vi "6.vi"   [LabVIEW 2017]
uses:
  <vilib>/myRIO/Instrument Drivers/Onboard IO/PWM/typedefs/PWM Reference.ctl
  <vilib>/myRIO/Common/Instrument Driver Framework/Utilities/typedefs/myRIO Generic Hardware Reference.ctl
  <vilib>/myRIO/Common/Instrument Driver Framework/Utilities/typedefs/Hardware Version Enum.ctl
  <vilib>/myRIO/Common/Instrument Driver Framework/Utilities/typedefs/myRIO v1.0 Reference.ctl
  <vilib>/myRIO/Common/Instrument Driver Framework/Utilities/typedefs/Generic FPGA Reference.ctl
  <vilib>/myRIO/Common/Instrument Driver Framework/myRIO v1.0/PWM/typedefs/PWM Channels Enum.ctl
  <vilib>/myRIO/Instrument Drivers/Onboard IO/PWM/typedefs/PWM Configuration.ctl
  <vilib>/userdefined/High Color/nirio_resource_hc.ctl
  <vilib>/myRIO/Common/Instrument Driver Framework/Utilities/vis/Is FPGA Ref Available.vi
  <vilib>/myRIO/Common/Instrument Driver Framework/myRIO v1.0/PWM/vis/myRIO v1.1 Open PWM.vi
  <vilib>/myRIO/Instrument Drivers/Onboard IO/PWM/vis/Set Duty Cycle and Frequency.vi
  <vilib>/myRIO/Common/Instrument Driver Framework/Utilities/vis/Validate Channels.vi
  <vilib>/myRIO/Common/Instrument Driver Framework/myRIO v1.0/PWM/vis/myRIO v1.0 Reserve PWM.vi
  <vilib>/myRIO/Common/Instrument Driver Framework/myRIO v1.0/PWM/vis/myRIO v1.0 Build MUX Configuration PWM.vi
  <vilib>/myRIO/Common/Instrument Driver Framework/myRIO v1.0/Resource Manager/vis/myRIO v1.0 Reserve Channel List.vi
  <vilib>/myRIO/Common/Instrument Driver Framework/myRIO v1.0/Resource Manager/vis/myRIO v1.0 Create Configuration List.vi
  <vilib>/myRIO/Common/Instrument Driver Framework/myRIO v1.0/Resource Manager/vis/myRIO v1.0 Reserve Channel.vi
  <vilib>/myRIO/Common/Instrument Driver Framework/myRIO v1.0/Resource Manager/vis/myRIO v1.0 Unreserve Channel.vi
  <vilib>/myRIO/Common/Instrument Driver Framework/myRIO v1.0/Resource Manager/vis/myRIO v1.0 Build Mutex Name.vi
  <vilib>/Utility/VariantDataType/GetNumericInfo.vi
  <vilib>/Utility/error.llb/Error Cluster From Error Code.vi
  <vilib>/myRIO/Common/Instrument Driver Framework/myRIO v1.0/myRIO v1.1 Open.vi
  <vilib>/myRIO/Common/Instrument Driver Framework/Utilities/vis/IO Manager.vi
  <vilib>/myRIO/Common/Instrument Driver Framework/Utilities/vis/Configuration Manager.vi
  <vilib>/myRIO/Common/Instrument Driver Framework/myRIO v1.0/Resource Manager/vis/myRIO v1.0 Configure IO.vi
  <vilib>/myRIO/Common/Instrument Driver Framework/myRIO v1.0/myRIO v1.0 Close.vi
  <vilib>/myRIO/Common/Instrument Driver Framework/myRIO v1.0/PWM/vis/myRIO v1.0 Write PWM.vi
  <vilib>/myRIO/Express VI/Onboard IO/PWM/PWM Express VI.xnode
  <vilib>/myRIO/Instrument Drivers/Onboard IO/PWM/vis/myRIO PWM Open.xnode
  <vilib>/myRIO/Instrument Drivers/Onboard IO/PWM/PWM.lvlib
types:
  T1 = typedef "PWM.lvlib/PWM Reference.ctl" = cluster{"myRIO Reference":T2, "PWM Channels Enum":T6, "PWM Configuration":T7}
  T2 = typedef "myRIO Generic Hardware Reference.ctl" = cluster{"myRIO Model":T3, "myRIO Hardware Reference":T4}
  T3 = typedef "Hardware Version Enum.ctl" = enum16{"Unknown", "myRIO-1900", "myRIO-1950", "roboRIO", "NI ELVIS RIO CM"}
  T4 = typedef "myRIO v1.0 Reference.ctl" = cluster{"Generic FPGA Reference":T5, "Allow multiple opens":bool}
  T5 = typedef "Generic FPGA Reference.ctl" = refnum<k20>
  T6 = typedef "PWM Channels Enum.ctl" = enum16{"Not Connected", "C/PWM0", "C/PWM1", "A/PWM0", "A/PWM1", "A/PWM2", "B/PWM0", "B/PWM1", "B/PWM2", "PWM/PWM0", "PWM/PWM1", "PWM/PWM2", "PWM/PWM3", "PWM/PWM4", "PWM/PWM5", "PWM/PWM6", "PWM/PWM7", "PWM/PWM8", "PWM/PWM9"}
  T7 = typedef "PWM.lvlib/PWM Configuration.ctl" = cluster{"Frequency":dbl, "Duty Cycle":dbl}
  T8 = typedef "nirio_resource_hc.ctl" = tag
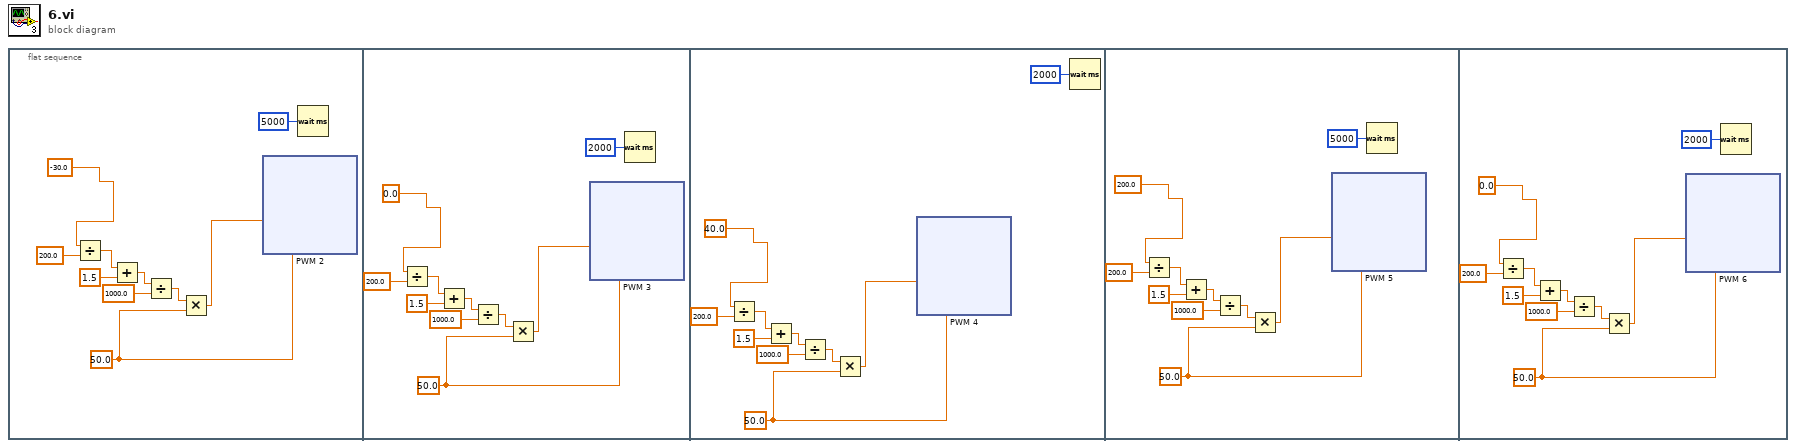
[diagram p0: block diagram]
diagram:
  n1 = flat-sequence {
    frame #0 {
      w6 = 50.0 ("Frequency [Hz]")
      n2 = Divide(x=-30.0, y=200.0) -> (x/y=w9:dbl)
      n3 = Add(x=w9, y=1.5) -> (x+y=w8:dbl)
      n4 = Divide(x=w8, y=1000.0) -> (x/y=w7:dbl)
      n5 = Multiply(x=w7, y=w6) -> (x*y=w10:dbl)
      n6 = xnode "PWM 2"("Duty Cycle"=w10, "Frequency [Hz]"=w6) -> ()  [unwired: 1 in, 1 out]
      n7 = Wait (ms)(milliseconds to wait=u32 5000) -> ()  [unwired: 1 out]
    }
    frame #1 {
      w51 = 50.0 ("Frequency [Hz]")
      n8 = Divide(x=0.0, y=200.0) -> (x/y=w54:dbl)
      n9 = Add(x=w54, y=1.5) -> (x+y=w53:dbl)
      n10 = Divide(x=w53, y=1000.0) -> (x/y=w52:dbl)
      n11 = Multiply(x=w52, y=w51) -> (x*y=w55:dbl)
      n12 = xnode "PWM 3"("Duty Cycle"=w55, "Frequency [Hz]"=w51) -> ()  [unwired: 1 in, 1 out]
      n13 = Wait (ms)(milliseconds to wait=u32 2000) -> ()  [unwired: 1 out]
    }
    frame #2 {
      w96 = 50.0 ("Frequency [Hz]")
      n14 = Divide(x=40.0, y=200.0) -> (x/y=w99:dbl)
      n15 = Add(x=w99, y=1.5) -> (x+y=w98:dbl)
      n16 = Divide(x=w98, y=1000.0) -> (x/y=w97:dbl)
      n17 = Multiply(x=w97, y=w96) -> (x*y=w100:dbl)
      n18 = xnode "PWM 4"("Duty Cycle"=w100, "Frequency [Hz]"=w96) -> ()  [unwired: 1 in, 1 out]
      n19 = Wait (ms)(milliseconds to wait=u32 2000) -> ()  [unwired: 1 out]
    }
    frame #3 {
      w141 = 50.0 ("Frequency [Hz]")
      n20 = Divide(x=200.0, y=200.0) -> (x/y=w144:dbl)
      n21 = Add(x=w144, y=1.5) -> (x+y=w143:dbl)
      n22 = Divide(x=w143, y=1000.0) -> (x/y=w142:dbl)
      n23 = Multiply(x=w142, y=w141) -> (x*y=w145:dbl)
      n24 = xnode "PWM 5"("Duty Cycle"=w145, "Frequency [Hz]"=w141) -> ()  [unwired: 1 in, 1 out]
      n25 = Wait (ms)(milliseconds to wait=u32 5000) -> ()  [unwired: 1 out]
    }
    frame #4 {
      w186 = 50.0 ("Frequency [Hz]")
      n26 = Divide(x=0.0, y=200.0) -> (x/y=w189:dbl)
      n27 = Add(x=w189, y=1.5) -> (x+y=w188:dbl)
      n28 = Divide(x=w188, y=1000.0) -> (x/y=w187:dbl)
      n29 = Multiply(x=w187, y=w186) -> (x*y=w190:dbl)
      n30 = xnode "PWM 6"("Duty Cycle"=w190, "Frequency [Hz]"=w186) -> ()  [unwired: 1 in, 1 out]
      n31 = Wait (ms)(milliseconds to wait=u32 2000) -> ()  [unwired: 1 out]
    }
  }
